vi "signed area.vi"(10 "Y":dbl[](array[numeric]), 11 "X":dbl[](array[numeric])) -> (3 "signed area":dbl)   [LabVIEW 2017]
uses:
  <vilib>/Analysis/NI_AALPro.lvlib
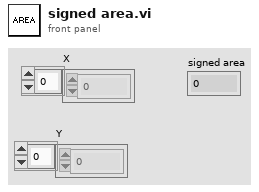
[diagram p1: front panel]
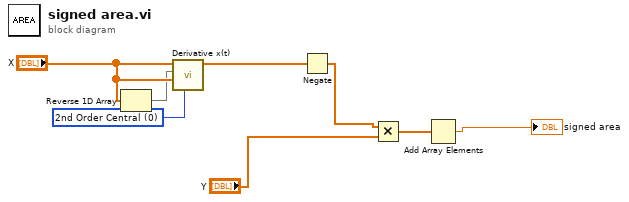
[diagram p0: block diagram]
diagram:
  w6 = u16 0 items=["2nd Order Central", "4th Order Central", "Forward", "Backward"] ("method")
  n1 = Reverse 1D Array(array="X") -> (reversed array=w7:dbl[])
  n2 = call <vilib>:"Derivative x(t).vi"("method"=w6, "Final Condition"="X", "Initial Condition"=w7, "X"="X") -> ("dX/dt"=w5:dbl[])  [unwired: 6 in, 1 out]
  n3 = Negate(x=w5) -> (-x=w4:dbl[])
  n4 = Multiply(x=w4, y="Y") -> (x*y=w2:dbl[])
  n5 = Add Array Elements(numeric array=w2) -> (sum=→"signed area":dbl)
